vi "Pre Launch Init.vi"(11 "UI Actor in":refnum<class "UI Actor.lvclass">) -> (0 "error out":errorcluster, 3 "UI Actor out":refnum<class "UI Actor.lvclass">)   [LabVIEW 2020, in "UI Actor.lvlib" / "UI Actor.lvclass"]
doc: "(<B>Filename</B>: Actor Framework.lvlib:Actor.lvclass:Pre Launch Init.vi)\n\nDefines behavior that occurs after the Launch Nested Actor method is invoked but before the actor's Actor Core method begins running.\n\nBy default, this method does nothing. A descendant class may override it to define behavior."
uses:
  UI Actor.lvclass
  UI Actor.lvclass/UI Actor.ctl
  <vilib>/ActorFramework/Actor/Actor.lvclass
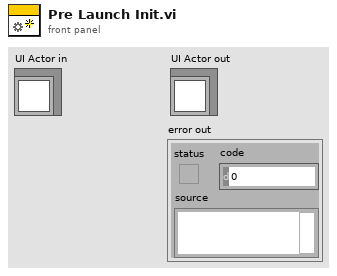
[diagram p1: front panel]
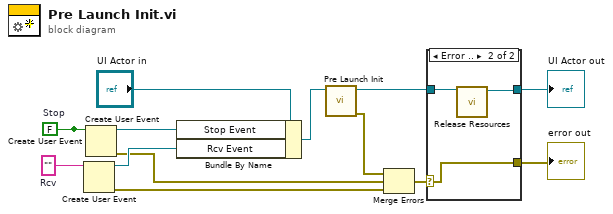
[diagram p0: block diagram]
diagram:
  w13 = ""  # Rcv
  w1 = FALSE  # Stop
  n1 = Create User Event(user event datatype=w13) -> (user event=w9:refnum<user-event>, error out=w2:errorcluster)  [unwired: 1 in]
  n2 = Create User Event(user event datatype=w1) -> (user event=w10:refnum<user-event>, error out=w3:errorcluster)  [unwired: 1 in]
  n3 = Create User Event(user event datatype=w1) -> ()  [unwired: 1 in, 2 out]
  n4 = Bundle By Name(cluster="UI Actor in", "Stop Event"=w10, "Rcv Event"=w9) -> (w11:refnum<class "UI Actor.lvclass">)
  n5 = call-parent "Pre Launch Init.vi"("Actor in"=w11) -> ("error out"=w4:errorcluster, "Actor out"=w6:refnum<class "UI Actor.lvclass">)  [unwired: 9 in]
  n6 = Merge Errors(w4, w3, w2) -> (w5:errorcluster)
  n7 = case shown="Error .." w5 {
    selector: w5 -> [w15 w16]
    tunnel: [w15 w16] -> w8
    tunnel: [w14 w17] -> w7
    tunnel: w6 -> [w14 w18]
    frame No Error {
    }
    frame Error {
      n8 = call "Release Resources.vi"("UI Actor in"=w18) -> ("UI Actor out"=w17:refnum<class "UI Actor.lvclass">)  [unwired: 10 in]
    }
  }
  "error out" <- w8
  "UI Actor out" <- w7
